vi "Result.Test Result to SFC1.vi"(8 "error in":errorcluster, 9 "Test Result":T1={"#attributes"={"Version"="MTE_1.0.0"}, "Station"={"Name"="", "PN"="", "SN"="", "Rev"="", "PC Name"="", "Location"="", "HW_Config"={"HW_Item"=[]}, "SW_Config"={"SW_Item"=[]}}, "Test Run"={"Operator"="", "Start Time"=timestamp(0 s since 1904-01-01), "Duration(s)"=0.0, "Mode"="", "Comment"="", "ProcessStep"=""}, "Test Sequence"={"Name"="", "Config"={"Config_Item"=[]}}, "UUTs"={"UUT"=[]}} {"UUTs"."UUT"."Measurements"."Measurement"."Status" items=["LOG", "PASS", "FAIL", "ERROR"]}, 10 "File Name":string, 11 "Dir":path) -> (0 "error out":errorcluster, 3 "Report Path":path)   [LabVIEW 2019]
uses:
  Result XML/TestResult.FullResultData.ctl
  Result XML/TestResult.Station Info.ctl
  Result XML/TestResult.HW Item.ctl
  Result XML/TestResult.SW Item.ctl
  Result XML/TestResult.Test Run Info.ctl
  Result XML/TestResult.Test Info.ctl
  Result XML/TestResult.UUT Result.ctl
  Result XML/TestResult.Symptom.ctl
  Result XML/TestResult.Symptom.State.ctl
  Result.Measurement Item.ctl
  Result.Measurement and Attribute Item Status.ctl
  Result XML/TestResult.UUTInfo.ctl
  <vilib>/KATE/Files/File Utils.lvlib
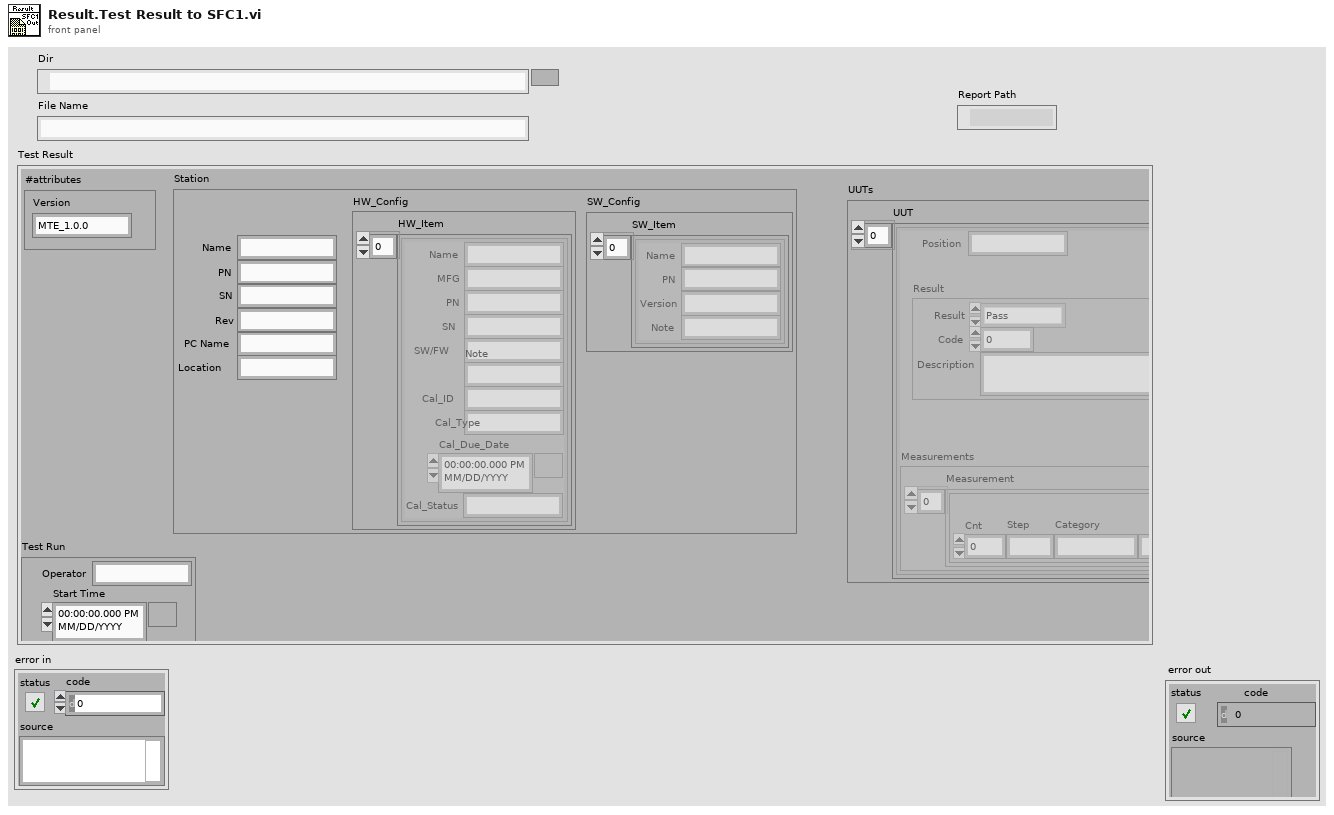
[diagram p1: front panel]
types:
  T1 = typedef "TestResult.FullResultData.ctl" = cluster{"#attributes":cluster{"Version":string}, "Station":T2, "Test Run":T5, "Test Sequence":T6, "UUTs":cluster{"UUT":T7[]}}
  T2 = typedef "TestResult.Station Info.ctl" = cluster{"Name":string, "PN":string, "SN":string, "Rev":string, "PC Name":string, "Location":string, "HW_Config":cluster{"HW_Item":T3[]}, "SW_Config":cluster{"SW_Item":T4[]}}
  T3 = typedef "TestResult.HW Item.ctl" = cluster{"Name":string, "MFG":string, "PN":string, "SN":string, "SW/FW":string, "Note":string, "Cal_ID":string, "Cal_Type":string, "Cal_Due_Date":timestamp, "Cal_Status":string}
  T4 = typedef "TestResult.SW Item.ctl" = cluster{"Name":string, "PN":string, "Version":string, "Note":string}
  T5 = typedef "TestResult.Test Run Info.ctl" = cluster{"Operator":string, "Start Time":timestamp, "Duration(s)":dbl, "Mode":string, "Comment":string, "ProcessStep":string}
  T6 = typedef "TestResult.Test Info.ctl" = cluster{"Name":string, "Config":cluster{"Config_Item":cluster{"Name":string, "Value":string}[]}}
  T7 = typedef "TestResult.UUT Result.ctl" = cluster{"Position":string, "Result":T8, "Measurements":cluster{"Measurement":T10[]}, "UUTInfo":T12}
  T8 = typedef "TestResult.Symptom.ctl" = cluster{"Result":T9, "Code":i32, "Description":string}
  T9 = typedef "TestResult.Symptom.State.ctl" = enum16{"Pass", "Fail", "Error", "Aborted", "Completed", "Logged"}
  T10 = typedef "Result.Measurement Item.ctl" = cluster{"Cnt":i32, "Step":string, "Category":string, "Name":string, "Value":string, "Units":string, "LimType":string, "LL":string, "UL":string, "Status":T11, "Code":i32, "Desc":string, "Time":timestamp}
  T11 = typedef "Result.Measurement and Attribute Item Status.ctl" = i32
  T12 = typedef "TestResult.UUTInfo.ctl" = cluster{"Product":string, "Desc":string, "PN":string, "SN":string, "Lot":string, "DateCode":string, "AltID":string, "Revision":string, "Properties":cluster{"Property":cluster{"Name":string, "Value":string}[]}}
  T13 = enum16{"open", "replace", "create", "open or create", "replace or create", "replace or create with confirmation"}
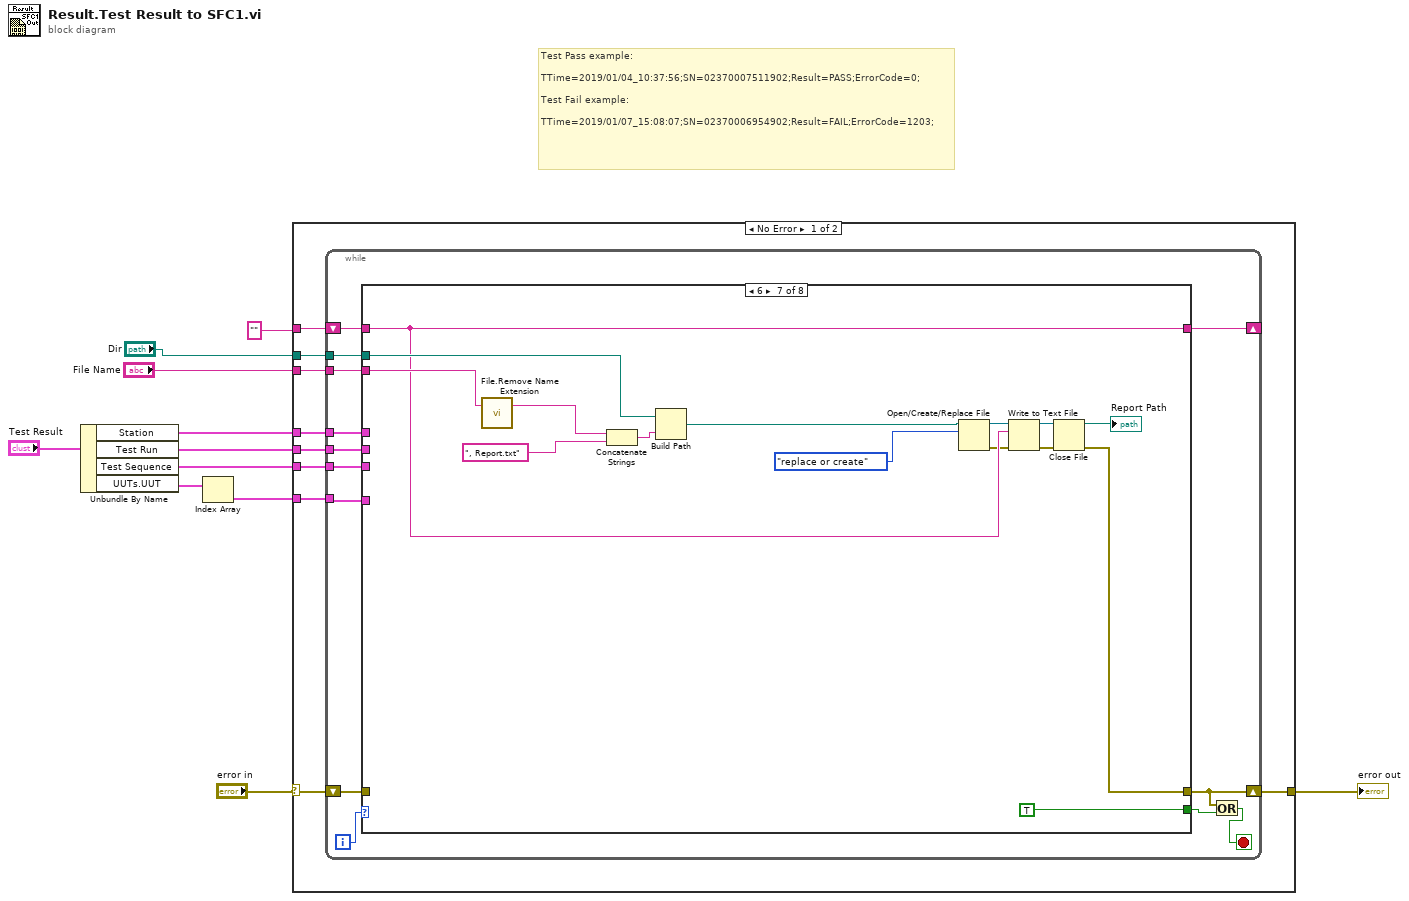
[diagram p0: block diagram]
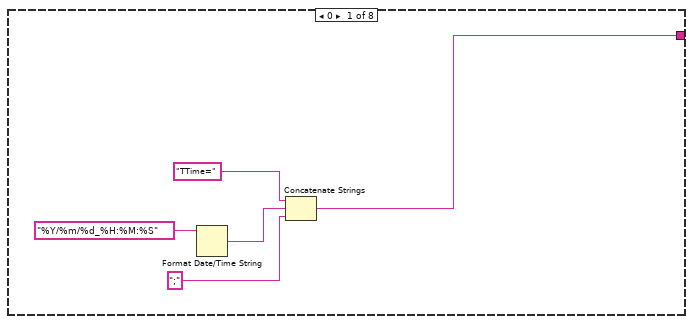
[diagram p2: hidden frame]
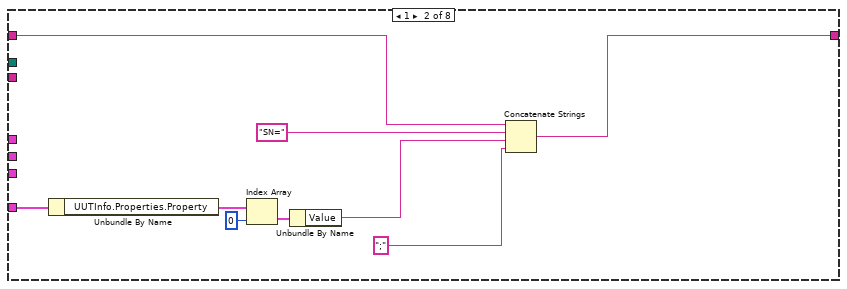
[diagram p3: hidden frame]
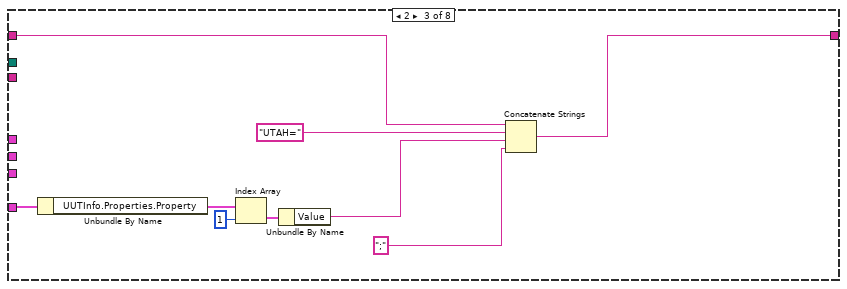
[diagram p4: hidden frame]
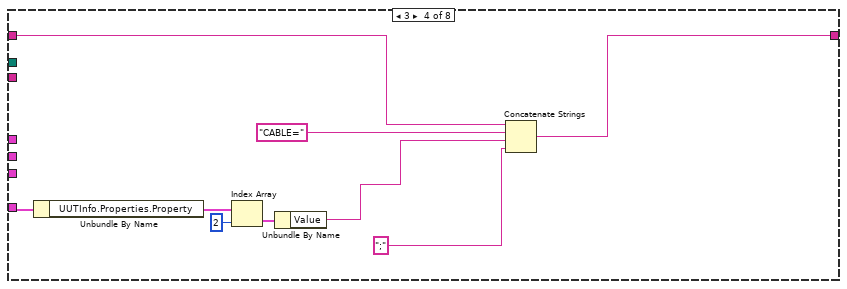
[diagram p5: hidden frame]
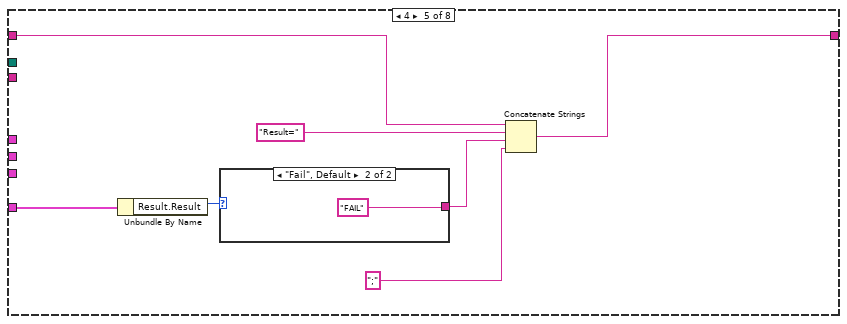
[diagram p6: hidden frame]
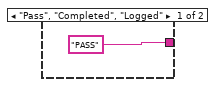
[diagram p7: hidden frame]
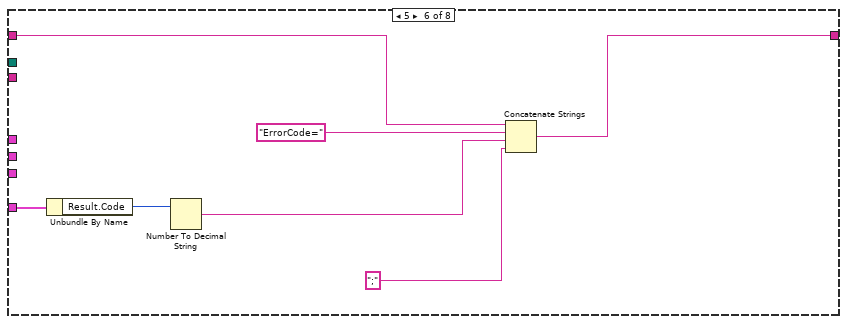
[diagram p8: hidden frame]
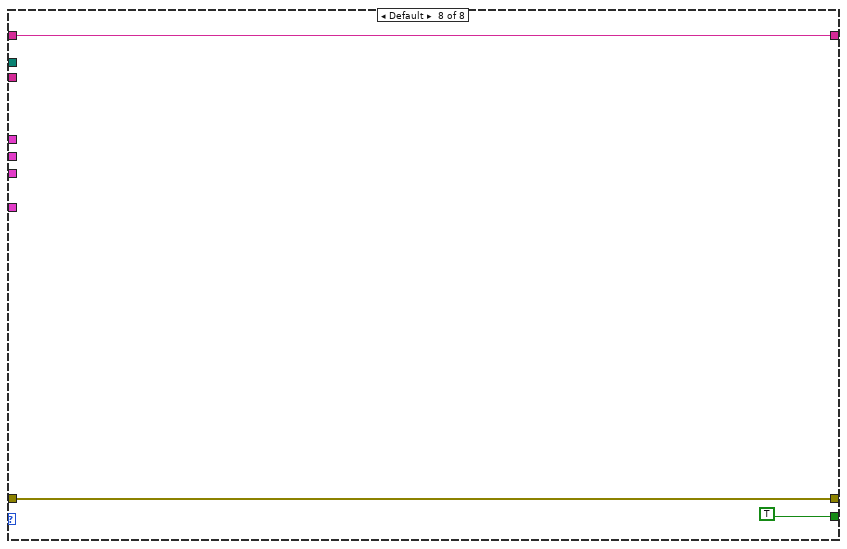
[diagram p9: hidden frame]
diagram:
  # "Test Pass example:\n\nTTime=2019/01/04_10:37:56;SN=02370007511902;Result=PASS;ErrorCode=0;\n\nTest Fail example:\n\nTTime=2019/01/07_15:08:07;SN=02370006954902;Result=FAIL;ErrorCode=1203;"
  n1 = Unbundle By Name("Test Result") -> ("Station"=w6:T2, "Test Run"=w5:T5, "Test Sequence"=w4:T6, "UUTs.UUT"=w8:T7[])
  n2 = Index Array(array=w8) -> (element=w7:T7)  [unwired: 1 in]
  n3 = case shown="No Error" "error in" {
    selector: "error in" -> [w19 w100]
    tunnel: [w20 w100] -> w11
    tunnel: w7 -> [w18 _]
    tunnel: w6 -> [w17 _]
    tunnel: w5 -> [w16 _]
    tunnel: w4 -> [w15 _]
    tunnel: "File Name" -> [w14 _]
    tunnel: "Dir" -> [w13 _]
    tunnel: "" -> [w12 _]
    frame No Error {
      n4 = while {
        shift-right: [w23] -> w20
        shift-left: w19 -> [w33]
        shift-right: [w26] -> _
        shift-left: w12 -> [w32]
        tunnel: w18 -> [w29]
        tunnel: w17 -> [w28]
        tunnel: w16 -> [w30]
        tunnel: w15 -> [w27]
        tunnel: w14 -> [w25]
        tunnel: w13 -> [w24]
        i -> [w31]
        stop <- w21 stop-if-true
        n5 = case shown="6" w31 {
          tunnel: [_ _ _ _ _ _ w90 w98] -> w23
          tunnel: w33 -> [_ _ _ _ _ _ _ w98]
          tunnel: w32 -> [_ w44 w53 w62 w69 w78 w87 w97]
          tunnel: [w34 w45 w54 w63 w70 w79 w87 w97] -> w26
          tunnel: w30 -> [_ _ _ _ _ _ _ _]
          tunnel: w29 -> [_ w43 w49 w58 w68 w77 _ _]
          tunnel: w28 -> [_ _ _ _ _ _ _ _]
          tunnel: w27 -> [_ _ _ _ _ _ _ _]
          tunnel: [_ _ _ _ _ _ TRUE TRUE] -> w22
          tunnel: w25 -> [_ _ _ _ _ _ w96 _]
          tunnel: w24 -> [_ _ _ _ _ _ w93 _]
          frame 0 {
            n6 = Format Date/Time String(time format string (%c)="%Y/%m/%d_%H:%M:%S") -> (date/time string=w36:string)  [unwired: 2 in]
            n7 = Concatenate Strings("TTime=", w36, ";") -> (w34:string)
          }
          frame 1 {
            n8 = Unbundle By Name(w43) -> ("UUTInfo.Properties.Property"=w42:cluster{"Name":string, "Value":string}[])
            n9 = Index Array(array=w42, index=0) -> (element=w40:cluster{"Name":string, "Value":string})
            n10 = Unbundle By Name(w40) -> ("Value"=w39:string)
            n11 = Concatenate Strings(w44, "SN=", w39, ";") -> (w45:string)
          }
          frame 2 {
            n12 = Unbundle By Name(w49) -> ("UUTInfo.Properties.Property"=w52:cluster{"Name":string, "Value":string}[])
            n13 = Index Array(array=w52, index=1) -> (element=w50:cluster{"Name":string, "Value":string})
            n14 = Unbundle By Name(w50) -> ("Value"=w48:string)
            n15 = Concatenate Strings(w53, "UTAH=", w48, ";") -> (w54:string)
          }
          frame 3 {
            n16 = Unbundle By Name(w58) -> ("UUTInfo.Properties.Property"=w61:cluster{"Name":string, "Value":string}[])
            n17 = Index Array(array=w61, index=2) -> (element=w59:cluster{"Name":string, "Value":string})
            n18 = Unbundle By Name(w59) -> ("Value"=w57:string)
            n19 = Concatenate Strings(w62, "CABLE=", w57, ";") -> (w63:string)
          }
          frame 4 {
            n20 = Unbundle By Name(w68) -> ("Result.Result"=w67:T9)
            n21 = case shown="\"Fail\", Default" w67 {
              tunnel: ["PASS" "FAIL"] -> w66
              frame "Pass", "Completed", "Logged" {
              }
              frame "Fail", Default {
              }
            }
            n22 = Concatenate Strings(w69, "Result=", w66, ";") -> (w70:string)
          }
          frame 5 {
            n23 = Unbundle By Name(w77) -> ("Result.Code"=w76:i32)
            n24 = Number To Decimal String(number=w76) -> (decimal integer string=w75:string)  [unwired: 1 in]
            n25 = Concatenate Strings(w78, "ErrorCode=", w75, ";") -> (w79:string)
          }
          frame 6 {
            n26 = call <vilib>:"File.Remove Name Extension.vi"("File Name"=w96) -> ("Name Less Ext"=w89:string)  [unwired: 1 in, 1 out]
            n27 = Concatenate Strings(w89, ", Report.txt" ("string")) -> (w94:string)
            n28 = Build Path(base path=w93, name or relative path=w94) -> (appended path=w91:path)
            n29 = Open/Create/Replace File(file path (use dialog)=w91, operation (0:open)=T13."replace or create") -> (refnum out=w84:refnum<file>, error out=w85:errorcluster)  [unwired: 4 in, 1 out]
            n30 = Write to Text File(file (use dialog)=w84, text=w87, error in=w85) -> (refnum out=w83:refnum<file>, error out=w86:errorcluster)  [unwired: 1 in, 1 out]
            n31 = Close File(refnum=w83, error in=w86) -> (path=→"Report Path":path, error out=w90:errorcluster)
          }
          frame Default {
          }
        }
        n32 = Or(x=w23, y=w22) -> (x .or. y?=w21:bool)
      }
    }
    frame Error {
    }
  }
  "error out" <- w11
